vi "PWM Write Port.vi"(0 "Arduino Resource":T1={"VISA resource"="", "Board Type"=enum."Arduino Uno", "Connection Type"=enum."USB / Serial", "Bytes Per Packet (15)"=15}, 1 "PWM Pins":u8[](array[numeric]), 5 "PWM 0 (0-255)":u8, 7 "PWM 1 (0-255)":u8, 9 "PWM 2 (0-255)":u8, 11 "error in":errorcluster) -> (4 "Arduino Resource":T1={"VISA resource"="", "Board Type"=enum."Arduino Uno", "Connection Type"=enum."USB / Serial", "Bytes Per Packet (15)"=15}, 8 "PWM Pins":u8[](array[numeric]), 15 "error out":errorcluster)   [LabVIEW 2011, in "LabVIEW Interface for Arduino.lvlib"]
doc: "Write specified PWM values to 3 PWM pins on the Arduino. The pins must first be configured for PWM using the PWM Configure Port VI."
uses:
  LabVIEW Interface for Arduino.lvlib
  Private/Type Defs/Arduino Resource.ctl
  Private/Type Defs/Board Type.ctl
  Private/Type Defs/Command.ctl
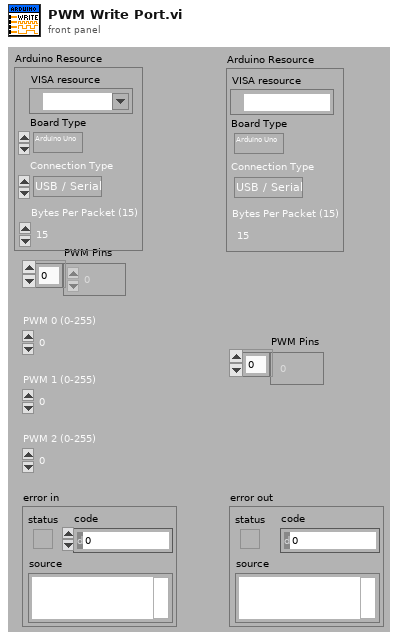
[diagram p1: front panel]
types:
  T1 = typedef "LabVIEW Interface for Arduino.lvlib/Arduino Resource.ctl" = cluster{"VISA resource":refnum<visa-resource-name>, "Board Type":T2, "Connection Type":enum8{"USB / Serial"}, "Bytes Per Packet (15)":u8}
  T2 = typedef "LabVIEW Interface for Arduino.lvlib/Board Type.ctl" = enum16{"Arduino Uno", "Dimuelanove w/Atmega 328", "Mega 2560", "Chipkit Uno32", "Chipkit Max32"}
  T3 = typedef "LabVIEW Interface for Arduino.lvlib/Command.ctl" = enum8{"setArduinoMode", "flushSerial", "setPinMode", "digitalWritePin", "digitalWritePort", "tone", "digitalReadPin", "digitalReadPort", "analogReadPin", "analogReadPort", "pwmWritePin", "pwmWritePort", "sevenSegment_Configure", "sevenSegment_Write", "I2C Init", "I2C Write", "I2C Read", "SPI Init", "SPI Set Bit Order", "SPI Set Clock Divider", "SPI Set Data Mode", "SPI Send / Receive", "SPI Close", "Servo Set Num Servos", "Servo Config Servo", "Servo Write Angle", "Servo Read Angle", "Servo Write Pulse Width", "Servo Read Pulse Width", "Servo Detach", "LCD Init", "LCD Set Size", "LCD Set Cursor Mode", "LCD Clear", "LCD Set Cursor Position", "LCD Print", "LCD Display Power", "LCD Scroll Display", "LCD Autoscroll", "LCD Print Direction", "LCD Create Custom Char", "LCD Print Custom Char", "contAcqOn", "contAcqOff", "getFirmwareVersion", "FiniteSampleStart"}
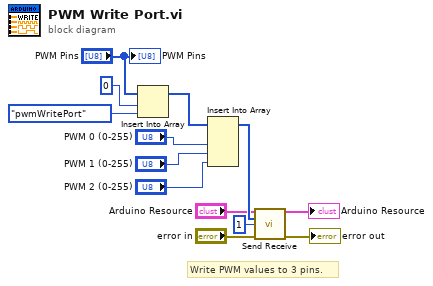
[diagram p0: block diagram]
diagram:
  # "Write PWM values to 3 pins."
  n1 = Insert Into Array(array="PWM Pins", index=0, new element=Command."pwmWritePort" ("Command")) -> (w10:u8[])
  n2 = Insert Into Array(array=w10, new element #1="PWM 0 (0-255)", new element #2="PWM 1 (0-255)", new element #3="PWM 2 (0-255)") -> (w6:u8[])  [unwired: 1 in]
  n3 = call "Send Receive.vi"("Arduino Resource"="Arduino Resource", "Data"=w6, "Bytes To Read (0)"=u32 1, "error in"="error in") -> ("Arduino Resource"=→"Arduino Resource":T1, "error out"=→"error out":errorcluster)  [unwired: 9 in, 1 out]
  "PWM Pins" <- "PWM Pins"
